vi "Command.vi"(8 "error in (no error)":errorcluster, 10 "command":string, 11 "Lotis in":refnum<class "PL Lotis TII LS.lvclass">) -> (0 "error out":errorcluster, 2 "response data":string, 3 "Lotis out":refnum<class "PL Lotis TII LS.lvclass">)   [LabVIEW 2015, in "PL Lotis TII LS.lvclass"]
doc: "Sends <b>command</b> to device and returns <b>response data</b>."
uses:
  PL Lotis TII LS.lvclass
  PL Lotis TII LS.lvclass/PL Lotis TII LS.ctl
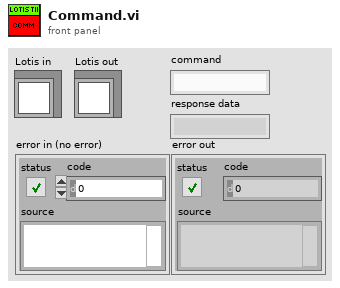
[diagram p1: front panel]
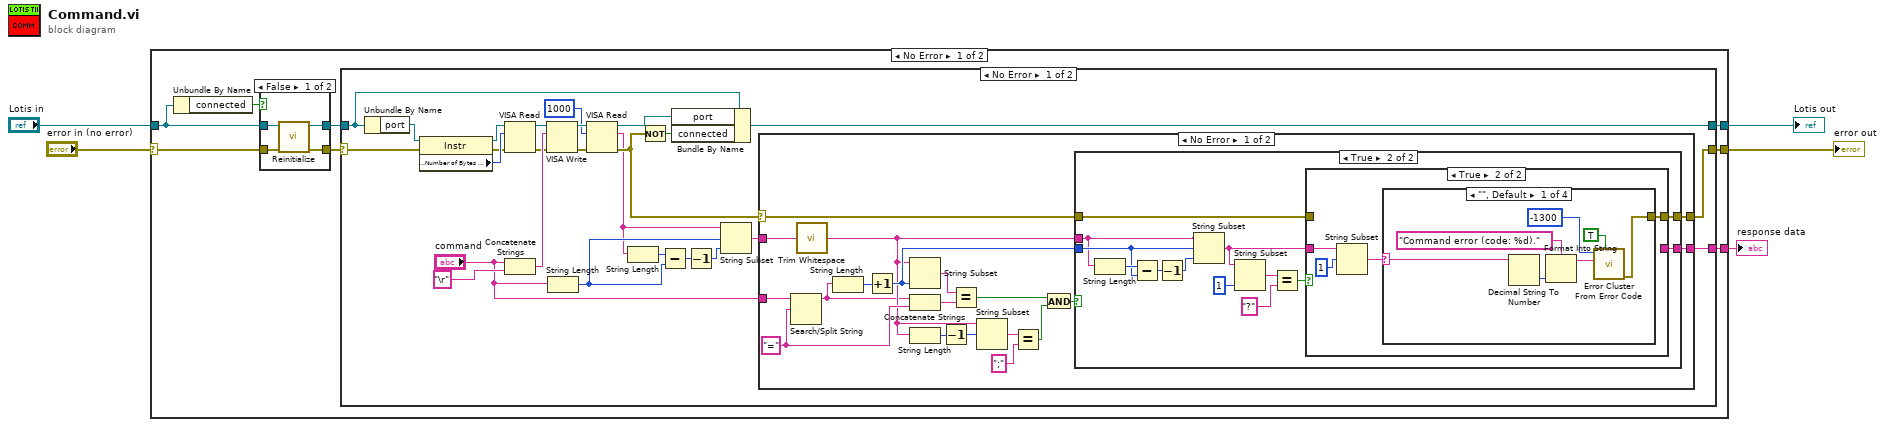
[diagram p0: block diagram]
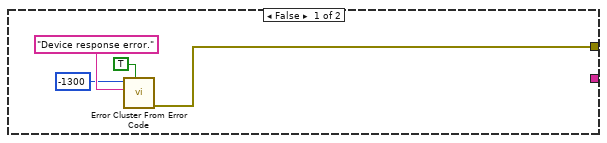
[diagram p2: hidden frame]
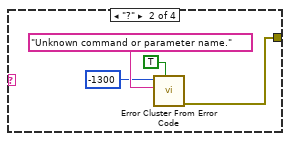
[diagram p4: hidden frame]
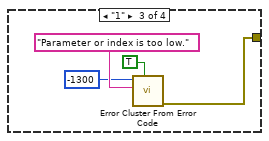
[diagram p5: hidden frame]
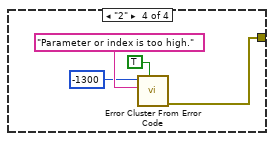
[diagram p6: hidden frame]
diagram:
  n1 = case shown="No Error" "error in (no error)" {
    selector: "error in (no error)" -> [w11 w111]
    tunnel: "Lotis in" -> [w12 w110]
    tunnel: [w8 w111] -> w2
    tunnel: [w7 w110] -> w3
    tunnel: [w6 _] -> w1
    frame No Error {
      n2 = Unbundle By Name(w12) -> ("connected"=w13:bool)
      n3 = case shown="False" w13 {
        tunnel: w12 -> [w107 w109]
        tunnel: w11 -> [w106 w108]
        tunnel: [w105 w109] -> w9
        tunnel: [w104 w108] -> w10
        frame False {
          n4 = call "Reinitialize.vi"("error in (no error)"=w106, "Lotis in"=w107) -> ("error out"=w104:errorcluster, "Lotis out"=w105:refnum<class "PL Lotis TII LS.lvclass">)  [unwired: 8 in]
        }
        frame True {
        }
      }
      n5 = case shown="No Error" w10 {
        selector: w10 -> [w22 w103]
        tunnel: w9 -> [w34 w102]
        tunnel: [w19 w103] -> w8
        tunnel: [w31 w102] -> w7
        tunnel: [w17 _] -> w6
        frame No Error {
          n6 = Unbundle By Name(w34) -> ("port"=w27:refnum<visa-resource-name>)
          n7 = property class="Instr"(reference=w27, error in=w22) -> (reference out=w26:refnum<visa-resource-name>, error out=w21:errorcluster, "Serial Settings:Number of Bytes at Serial Port"=w24:u32)
          n8 = VISA Read(VISA resource name=w26, byte count=w24, error in (no error)=w21) -> (VISA resource name out=w25:refnum<visa-resource-name>, error out=w23:errorcluster)  [unwired: 2 out]
          n9 = Concatenate Strings("command", "\r" ("string")) -> (w36:string)
          n10 = VISA Write(VISA resource name=w25, write buffer=w36, error in (no error)=w23) -> (VISA resource name out=w39:refnum<visa-resource-name>, error out=w38:errorcluster)  [unwired: 1 out]
          n11 = String Length(string="command") -> (length=w18:i32)
          n12 = VISA Read(VISA resource name=w39, byte count=u32 1000, error in (no error)=w38) -> (VISA resource name out=w33:refnum<visa-resource-name>, read buffer=w16:string, error out=w20:errorcluster)  [unwired: 1 out]
          n13 = String Length(string=w16) -> (length=w30:i32)
          n14 = Not(x=w20) -> (.not. x?=w32:bool)
          n15 = Subtract(x=w30, y=w18) -> (x-y=w29:i32)
          n16 = Bundle By Name(cluster=w34, "port"=w33, "connected"=w32) -> (w31:refnum<class "PL Lotis TII LS.lvclass">)
          n17 = Decrement(x=w29) -> (x-1=w28:i32)
          n18 = String Subset(string=w16, offset (0)=w18, length (rest)=w28) -> (substring=w15:string)
          n19 = case shown="No Error" w20 {
            selector: w20 -> [w49 w101]
            tunnel: [w48 w101] -> w19
            tunnel: [w46 _] -> w17
            tunnel: w15 -> [w45 _]
            tunnel: "command" -> [w44 _]
            frame No Error {
              w43 = "=" ("string")
              n20 = Search/Split String(string=w44, search string/char (-)=w43) -> (substring before match=w40:string)  [unwired: 1 in, 2 out]
              n21 = call <vilib>:"Trim Whitespace.vi"("string"=w45) -> ("trimmed string"=w42:string)  [unwired: 1 in]
              n22 = String Length(string=w40) -> (length=w41:i32)
              n23 = Increment(x=w41) -> (x+1=w47:i32)
              n24 = String Subset(string=w42, length (rest)=w47) -> (substring=w58:string)  [unwired: 1 in]
              n25 = Concatenate Strings(w40, w43) -> (w57:string)
              n26 = String Length(string=w42) -> (length=w56:i32)
              n27 = Decrement(x=w56) -> (x-1=w55:i32)
              n28 = Equal?(x=w58, y=w57) -> (x = y?=w52:bool)
              n29 = String Subset(string=w42, offset (0)=w55) -> (substring=w54:string)  [unwired: 1 in]
              n30 = Equal?(x=w54, y=";") -> (x = y?=w51:bool)
              n31 = And(x=w52, y=w51) -> (x .and. y?=w50:bool)
              n32 = case shown="True" w50 {
                tunnel: w49 -> [_ w67]
                tunnel: [w59 w66] -> w48
                tunnel: w42 -> [_ w63]
                tunnel: w47 -> [_ w74]
                tunnel: [_ w64] -> w46
                frame False {
                  n33 = call <vilib>:"Error Cluster From Error Code.vi"("show call chain? (False)"=TRUE, "error message (\"\")"="Device response error." ("format string"), "error code (0)"=-1300) -> ("error out"=w59:errorcluster)  [unwired: 6 in]
                }
                frame True {
                  n34 = String Length(string=w63) -> (length=w75:i32)
                  n35 = Subtract(x=w75, y=w74) -> (x-y=w73:i32)
                  n36 = Decrement(x=w73) -> (x-1=w72:i32)
                  n37 = String Subset(string=w63, offset (0)=w74, length (rest)=w72) -> (substring=w65:string)
                  n38 = String Subset(string=w65, length (rest)=1 ("length (rest)")) -> (substring=w70:string)  [unwired: 1 in]
                  n39 = Equal?(x=w70, y="?") -> (x = y?=w68:bool)
                  n40 = case shown="True" w68 {
                    tunnel: w67 -> [w77 _]
                    tunnel: [w77 w78] -> w66
                    tunnel: [w76 _] -> w64
                    tunnel: w65 -> [w76 w81]
                    frame False {
                    }
                    frame True {
                      n41 = String Subset(string=w81, offset (0)=1 ("length (rest)")) -> (substring=w79:string)  [unwired: 1 in]
                      n42 = case shown="\"\", Default" w79 {
                        selector: w79 -> [w83 _ _ _]
                        tunnel: [w82 w89 w93 w97] -> w78
                        frame "", Default {
                          n43 = Decimal String To Number(string=w83) -> (number=w88:i32)  [unwired: 2 in, 1 out]
                          n44 = Format Into String(format string="Command error (code: %d).", w88) -> (resulting string=w87:string)  [unwired: 2 in, 1 out]
                          n45 = call <vilib>:"Error Cluster From Error Code.vi"("show call chain? (False)"=TRUE, "error message (\"\")"=w87, "error code (0)"=-1300) -> ("error out"=w82:errorcluster)  [unwired: 6 in]
                        }
                        frame "?" {
                          n46 = call <vilib>:"Error Cluster From Error Code.vi"("show call chain? (False)"=TRUE, "error message (\"\")"="Unknown command or parameter name." ("format string"), "error code (0)"=-1300) -> ("error out"=w89:errorcluster)  [unwired: 6 in]
                        }
                        frame "1" {
                          n47 = call <vilib>:"Error Cluster From Error Code.vi"("show call chain? (False)"=TRUE, "error message (\"\")"="Parameter or index is too low." ("format string"), "error code (0)"=-1300) -> ("error out"=w93:errorcluster)  [unwired: 6 in]
                        }
                        frame "2" {
                          n48 = call <vilib>:"Error Cluster From Error Code.vi"("show call chain? (False)"=TRUE, "error message (\"\")"="Parameter or index is too high." ("format string"), "error code (0)"=-1300) -> ("error out"=w97:errorcluster)  [unwired: 6 in]
                        }
                      }
                    }
                  }
                }
              }
            }
            frame Error {
            }
          }
        }
        frame Error {
        }
      }
    }
    frame Error {
    }
  }
  "Lotis out" <- w3
  "response data" <- w1
  "error out" <- w2
